vi "ModelParameters.UpdateFromFile.vi"(9 "ModelParameterFiles":string[](array[string]), 10 "Target":string, 11 "GatewayIP":string) -> (0 "error out":errorcluster)   [LabVIEW 2013, in "MiscHelperVIs.lvlib"]
uses:
  MiscHelperVIs.lvlib
  NationalInstruments.VeriStand.ClientAPI
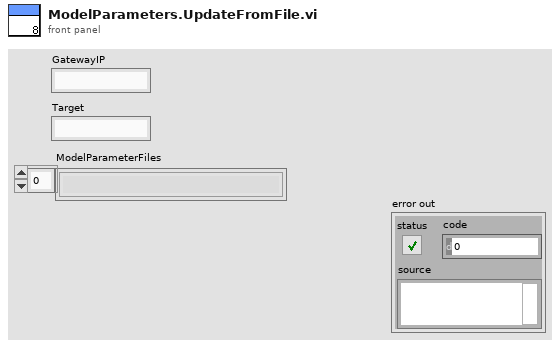
[diagram p1: front panel]
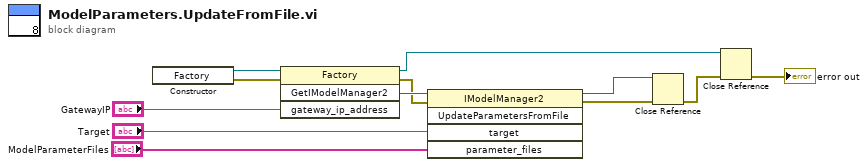
[diagram p0: block diagram]
diagram:
  n1 = constructor class="Factory"() -> (reference out=w12:refnum<k24>, error out=w11:errorcluster)  [unwired: 3 in, 1 out]
  n2 = invoke class="Factory" method="GetIModelManager2"(reference=w12, error in=w11, "gateway_ip_address"="GatewayIP") -> (reference out=w4:refnum<k24>, error out=w5:errorcluster, "GetIModelManager2"=w9:refnum<k24>)  [unwired: 1 in, 1 out]
  n3 = invoke class="IModelManager2" method="UpdateParametersFromFile"(reference=w9, error in=w5, "target"="Target", "parameter_files"="ModelParameterFiles") -> (reference out=w6:refnum<k24>, error out=w7:errorcluster)  [unwired: 1 in, 3 out]
  n4 = Close Reference(reference=w6, error in (no error)=w7) -> (error out=w3:errorcluster)
  n5 = Close Reference(reference=w4, error in (no error)=w3) -> (error out=→"error out":errorcluster)
